vi "Filter_subvi.vi"(1 "Filter Select":u16, 2 "Filter Order":i16(knob) scale=1.0..5.0, 3 "Filter Cut Off Frequency":dbl, 4 "Waveform":waveform(dbl)) -> (0 "Filtered Signal":dynamicdata(waveform))   [LabVIEW 2020]
uses:
  <vilib>/Analysis/3filter.llb/Filter Passband Type.ctl
  <vilib>/Analysis/3filter.llb/Butterworth Filter (DBL).vi
  <vilib>/Analysis/NI_AALBase.lvlib
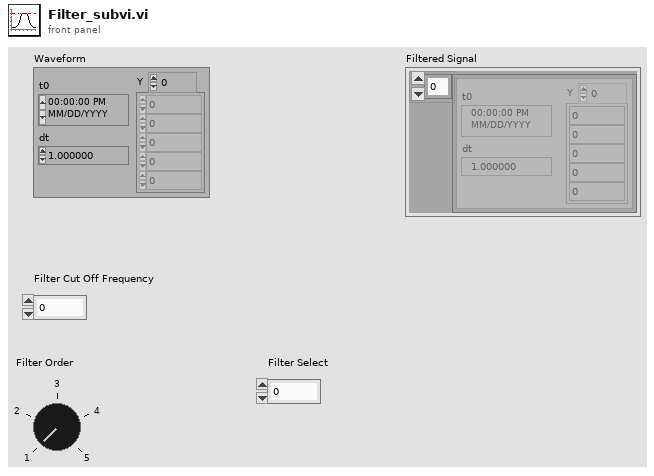
[diagram p1: front panel]
types:
  T1 = typedef "NI_AALBase.lvlib/Filter Passband Type.ctl" = enum32{"Lowpass", "Highpass", "Bandpass", "Bandstop"}
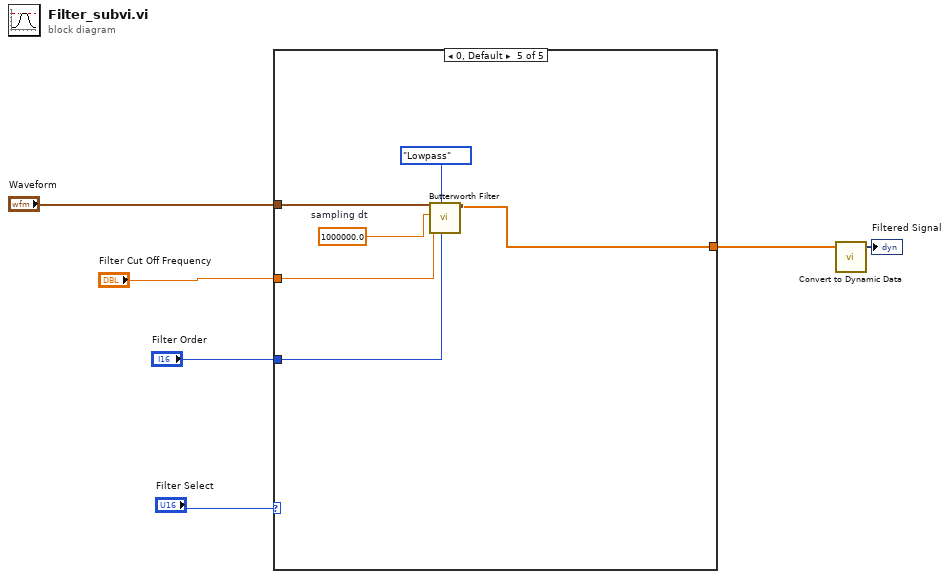
[diagram p0: block diagram]
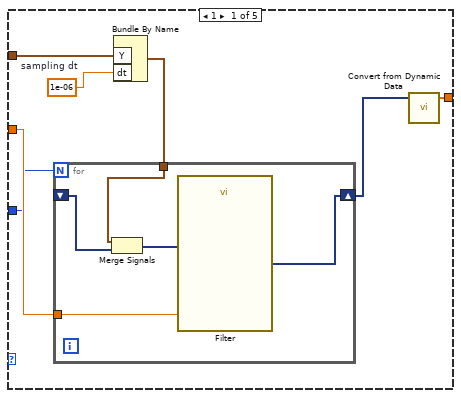
[diagram p2: hidden frame]
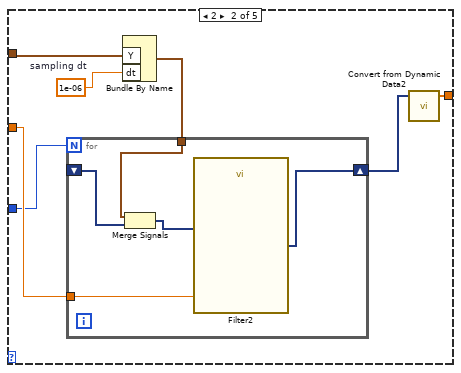
[diagram p3: hidden frame]
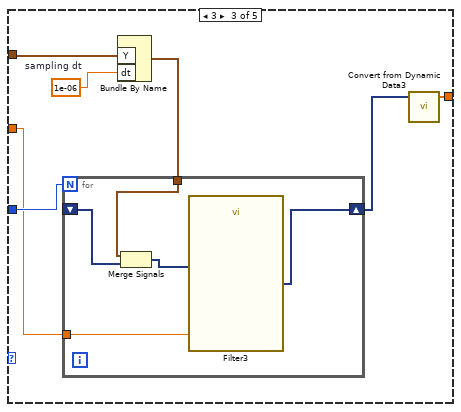
[diagram p4: hidden frame]
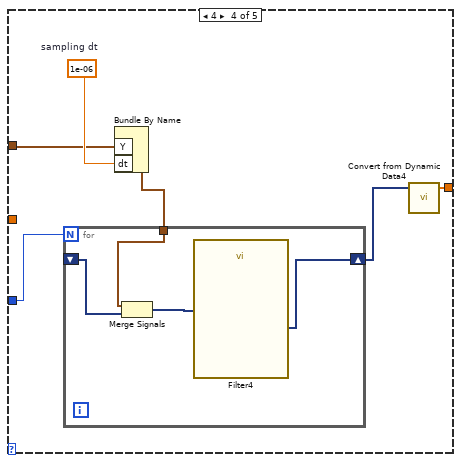
[diagram p5: hidden frame]
diagram:
  n1 = case shown="0, Default" "Filter Select" {
    tunnel: [w7 w19 w31 w43 w54] -> w2
    tunnel: "Filter Cut Off Frequency" -> [w11 w23 w34 _ w56]
    tunnel: "Filter Order" -> [w8 w20 w35 w46 w55]
    tunnel: "Waveform" -> [w12 w24 w36 w47 w58]
    frame 1 {
      w13 = 1e-06  # sampling dt
      n2 = Bundle By Name("Y"=w12, "dt"=w13) -> (w10:waveform(dbl))  [unwired: 1 in]
      n3 = for {
        N: w8 -> [_]
        shift-right: [w17] -> w9
        shift-left: _ -> [w14]
        tunnel: w11 -> [w18]
        tunnel: w10 -> [w15]
        n4 = Merge Signals(w15, w14) -> (w16:dynamicdata)
        n5 = call "Filter"("Lower Cut-Off"=w18, "Signal"=w16) -> ("Filtered Signal"=w17:dynamicdata)  [unwired: 8 in, 1 out]
      }
      n6 = call "Convert from Dynamic Data"("Dynamic Data Type"=w9) -> ("Array"=w7:dbl[])  [unwired: 3 in]
    }
    frame 2 {
      w25 = 1e-06  # sampling dt
      n7 = Bundle By Name("Y"=w24, "dt"=w25) -> (w22:waveform(dbl))  [unwired: 1 in]
      n8 = for {
        N: w20 -> [_]
        shift-right: [w26] -> w21
        shift-left: _ -> [w28]
        tunnel: w23 -> [w30]
        tunnel: w22 -> [w29]
        n9 = Merge Signals(w29, w28) -> (w27:dynamicdata)
        n10 = call "Filter2"("Lower Cut-Off"=w30, "Signal"=w27) -> ("Filtered Signal"=w26:dynamicdata)  [unwired: 8 in, 1 out]
      }
      n11 = call "Convert from Dynamic Data2"("Dynamic Data Type"=w21) -> ("Array"=w19:dbl[])  [unwired: 3 in]
    }
    frame 3 {
      w37 = 1e-06  # sampling dt
      n12 = Bundle By Name("Y"=w36, "dt"=w37) -> (w33:waveform(dbl))  [unwired: 1 in]
      n13 = for {
        N: w35 -> [_]
        shift-right: [w38] -> w32
        shift-left: _ -> [w40]
        tunnel: w34 -> [w42]
        tunnel: w33 -> [w41]
        n14 = Merge Signals(w41, w40) -> (w39:dynamicdata)
        n15 = call "Filter3"("Lower Cut-Off"=w42, "Signal"=w39) -> ("Filtered Signal"=w38:dynamicdata)  [unwired: 8 in, 1 out]
      }
      n16 = call "Convert from Dynamic Data3"("Dynamic Data Type"=w32) -> ("Array"=w31:dbl[])  [unwired: 3 in]
    }
    frame 4 {
      w48 = 1e-06  # sampling dt
      n17 = Bundle By Name("Y"=w47, "dt"=w48) -> (w45:waveform(dbl))  [unwired: 1 in]
      n18 = for {
        N: w46 -> [_]
        shift-right: [w51] -> w44
        shift-left: _ -> [w49]
        tunnel: w45 -> [w52]
        n19 = Merge Signals(w52, w49) -> (w50:dynamicdata)
        n20 = call "Filter4"("Signal"=w50) -> ("Filtered Signal"=w51:dynamicdata)  [unwired: 9 in, 1 out]
      }
      n21 = call "Convert from Dynamic Data4"("Dynamic Data Type"=w44) -> ("Array"=w43:dbl[])  [unwired: 3 in]
    }
    frame 0, Default {
      w57 = 1000000.0  # sampling dt
      n22 = call-poly <vilib>:"Butterworth Filter.vi"("order"=w55, "filter type"=Filter_Passband_Type."Lowpass", "low cutoff freq: fl"=w56, "sampling freq: fs"=w57, "X"=w58) -> ("Filtered X"=w54:dbl[])  [unwired: 3 in, 1 out]
    }
  }
  n23 = call "Convert to Dynamic Data"("Array"=w2) -> ("Dynamic Data Type"=→"Filtered Signal":dynamicdata)  [unwired: 3 in]
